vi "BufferedAverageFilter.vi"(7 "Buffer Size":i32, 11 "Signal":dbl) -> (3 "FilteredSignal":dbl)   [LabVIEW 2018]
doc: "Simple Low-Pass filter.\nAverages the last N samples."
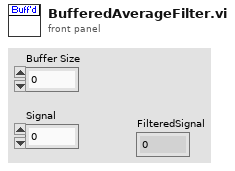
[diagram p1: front panel]
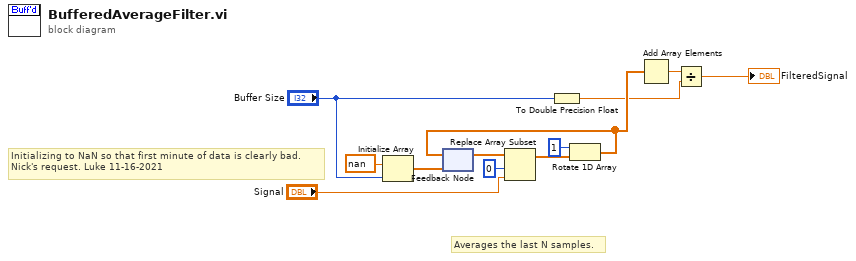
[diagram p0: block diagram]
diagram:
  # "Initializing to NaN so that first minute of data is clearly bad.\nNick's request. Luke 11-16-2021"
  # "Averages the last N samples."
  n1 = Initialize Array(nan, "Buffer Size") -> (w5:dbl[])
  n2 = feedback #1(w5) -> (w7:dbl[])
  n3 = Replace Array Subset(array=w7, new element="Signal", index=0) -> (w8:dbl[])
  n4 = To Double Precision Float(number="Buffer Size") -> (double precision float=w4:dbl)
  n5 = Rotate 1D Array(1:w8, 2:1 ("n")) -> (0:w10:dbl[])
  n6 = feedback-in #1(w10) -> ()
  n7 = Add Array Elements(numeric array=w10) -> (sum=w11:dbl)
  n8 = Divide(x=w11, y=w4) -> (x/y=→"FilteredSignal":dbl)
